vi "Set drive reset (after trip condition).vi"(4 "Drive address":T3=1 items=["0", "1", "2", "3", "4", "5", "6", "7", "8", "9", "10", "11", "12", "13", "14", "15", "16", "17", "18", "19", "20", "21", "22", "23", "24", "25", "26", "27", "28", "29", "30", "31", "32", "33", "34", "35", "36", "37", "38", "39", "40", "41", "42", "43", "44", "45", "46", "47", "48", "49", "50", "51", "52", "53", "54", "55", "56", "57", "58", "59", "60", "61", "62", "63"], 5 "COM port":refnum<visa-resource-name>) -> (1 "Modbus error cluster":T1={"Checksum ok"=FALSE, "Modbus exception code"=1, "Response from correct drive"=FALSE, "Comms error"={"status"=FALSE, "code"=0, "source"=""}} {"Modbus exception code" items=["None"=0, "Invalid function request"=1, "Invalid Modbus register address"=2, "Invalid / unauthorised data value"=3, "Device failure"=4, "Request accepted, wait"=5, "Drive busy"=6, "Request rejected"=7, "Memory parity error"=8, "Gateway path unavailable"=10, "Device failed to respond"=11]}, 2 "No errors":bool)   [LabVIEW 2020]
doc: "Modbus RTU for Invertek drives. Paul Nathan 21-JUN-2022."
uses:
  ctls/Drive address.ctl
  ctls/Register.ctl
  ctls/Exception codes.ctl
  ctls/Modbus error cluster.ctl
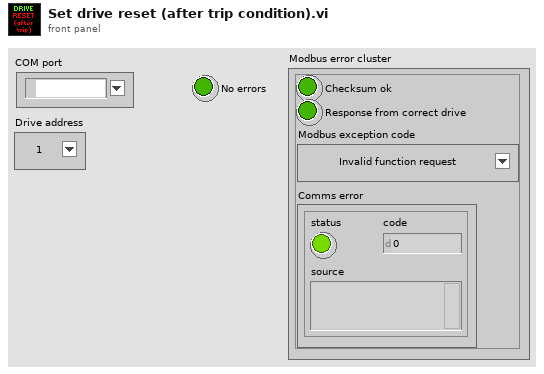
[diagram p1: front panel]
types:
  T1 = typedef "Modbus error cluster.ctl" = cluster{"Checksum ok":bool, "Modbus exception code":T2, "Response from correct drive":bool, "Comms error":errorcluster}
  T2 = typedef "Exception codes.ctl" = u8
  T3 = typedef "Drive address.ctl" = u8
  T4 = typedef "Register.ctl" = u16
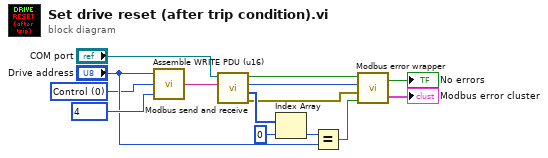
[diagram p0: block diagram]
diagram:
  w7 = T4 0 items=["Control"=0, "RPM set-point"=4, "Drive status"=5, "Output RPM"=6, "Motor current"=7, "Motor torque"=8, "Motor power"=9, "DC bus voltage"=22, "Drive power stage temperature"=23, "kWh meter"=31, "MWh meter"=32, "Running time - hours"=33, "Running time - seconds"=34, "Internal drive temperature"=38, "Motor RMS voltage"=42, "Extended drive status"=2000] ("Register")
  n1 = call "Assemble WRITE PDU (u16).vi"("u16 value"=u16 4, "Register"=w7, "Drive address"="Drive address") -> ("Ser out string"=w13:string)
  n2 = call "Modbus send and receive.vi"("Modbus telegram"=w13, "COM port"="COM port") -> ("Comms error"=w2:errorcluster, "Device response"=w11:u8[], "Modbus exception code"=w3:T2, "Checksum ok"=w4:bool)  [unwired: 2 in]
  n3 = Index Array(array=w11, index=0) -> (element=w9:u8)
  n4 = Equal?(x=w9, y="Drive address") -> (x = y?=w1:bool)
  n5 = call "Modbus error wrapper.vi"("Response from correct drive"=w1, "Comms error"=w2, "Modbus exception code"=w3, "Checksum ok"=w4) -> ("Modbus error cluster"=→"Modbus error cluster":T1, "No errors"=→"No errors":bool)
